vi "get_object_terminals.vi"(11 "object id":string) -> (0 "error out":errorcluster, 3 "Terminal Description":string)   [LabVIEW 2026]
doc: "Returns the Terminals Names and/or descriptions as a string as well as their Index to be used in other functions like connect objects."
uses:
  G-AI Core/G-AI Core.lvlib
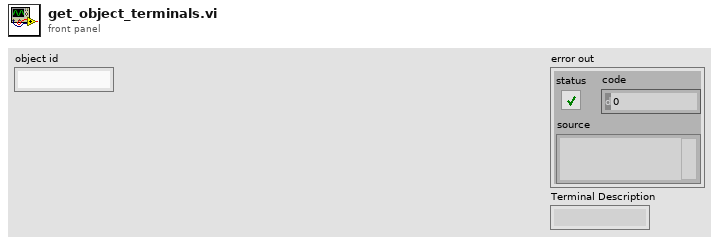
[diagram p1: front panel]
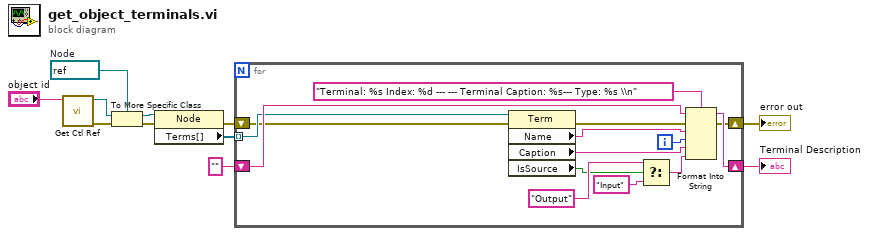
[diagram p0: block diagram]
diagram:
  w8 = refnum<vi> refnum  # Node
  n1 = call "Get Ctl Ref.vi"("ctl id"="object id") -> ("error out"=w2:errorcluster, "ctl ref"=w3:refnum<vi>)  [unwired: 9 in]
  n2 = To More Specific Class(target class=w8, reference=w3, error in=w2) -> (specific class reference=w7:refnum<vi>, error out=w6:errorcluster)
  n3 = property class="Node"(reference=w7, error in=w6) -> (error out=w11:errorcluster, "Terms[]"=w10:refnum<vi>[])  [unwired: 1 out]
  n4 = for {
    shift-right: [w24] -> w4
    shift-left: "" -> [w25]
    tunnel: w10 -> [w22] mode=indexing
    shift-right: [w12] -> w5
    shift-left: w11 -> [w21]
    i -> [w14]
    n5 = property class="Term"(reference=w22, error in=w21) -> (error out=w13:errorcluster, "Name"=w16:string, "Caption"=w15:string, "IsSource"=w19:bool)  [unwired: 1 out]
    n6 = Select(t="Output" ("input 4"), s=w19, f="Input" ("input 4")) -> (s? t:f=w18:string)
    n7 = Format Into String(format string="Terminal: %s Index: %d --- --- Terminal Caption: %s--- Type: %s \\n", initial string=w25, error in=w13, w16, w14, w15, w18) -> (resulting string=w24:string, error out=w12:errorcluster)
  }
  "error out" <- w5
  "Terminal Description" <- w4
